vi "Create RSAEncryptionPadding.vi"(8 "error in (no error)":errorcluster, 11 "Padding Mode":T1) -> (0 "error out":errorcluster, 3 "RSAEncryptionPadding":refnum<k24>)   [LabVIEW 2021, in "dotNET Crypto Asymmetric Encryption.lvlib"]
doc: "Creates an RSAEncryptionPadding object - ensure that the object is closed to avoid a reference leak."
uses:
  dotNET Crypto Asymmetric Encryption.lvlib
  RSAEncryptionPadding.ctl
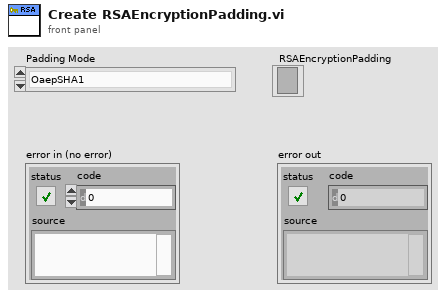
[diagram p1: front panel]
types:
  T1 = typedef "dotNET Crypto Asymmetric Encryption.lvlib/RSAEncryptionPadding.ctl" = enum16{"OaepSHA1", "OaepSHA256", "OaepSHA384", "OaepSHA512", "Pkcs1"}
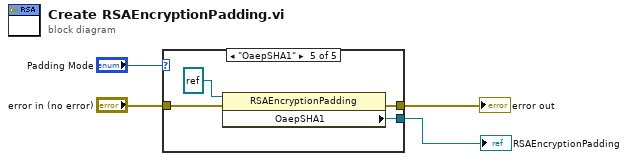
[diagram p0: block diagram]
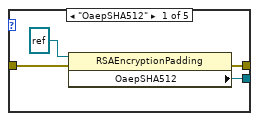
[diagram p2: hidden frame]
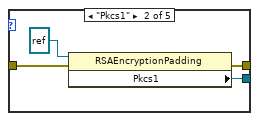
[diagram p3: hidden frame]
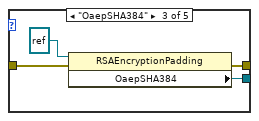
[diagram p4: hidden frame]
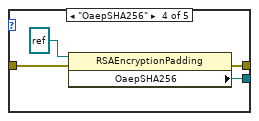
[diagram p5: hidden frame]
diagram:
  n1 = case shown="\"OaepSHA1\"" "Padding Mode" {
    tunnel: [w7 w11 w15 w19 w23] -> w1
    tunnel: "error in (no error)" -> [w6 w10 w13 w18 w22]
    tunnel: [w5 w9 w14 w17 w21] -> w3
    frame "OaepSHA512" {
      n2 = property class="RSAEncryptionPadding"(reference=refnum<k24> refnum ("padding"), error in=w6) -> (error out=w5:errorcluster, "OaepSHA512"=w7:refnum<k24>)  [unwired: 1 out]
    }
    frame "Pkcs1" {
      n3 = property class="RSAEncryptionPadding"(reference=refnum<k24> refnum ("padding"), error in=w10) -> (error out=w9:errorcluster, "Pkcs1"=w11:refnum<k24>)  [unwired: 1 out]
    }
    frame "OaepSHA384" {
      n4 = property class="RSAEncryptionPadding"(reference=refnum<k24> refnum ("padding"), error in=w13) -> (error out=w14:errorcluster, "OaepSHA384"=w15:refnum<k24>)  [unwired: 1 out]
    }
    frame "OaepSHA256" {
      n5 = property class="RSAEncryptionPadding"(reference=refnum<k24> refnum ("padding"), error in=w18) -> (error out=w17:errorcluster, "OaepSHA256"=w19:refnum<k24>)  [unwired: 1 out]
    }
    frame "OaepSHA1" {
      n6 = property class="RSAEncryptionPadding"(reference=refnum<k24> refnum ("padding"), error in=w22) -> (error out=w21:errorcluster, "OaepSHA1"=w23:refnum<k24>)  [unwired: 1 out]
    }
  }
  "error out" <- w3
  "RSAEncryptionPadding" <- w1
